vi "Initialize.vi"(8 "error in (no error)":errorcluster, 11 "Coins in":refnum<class "Coins.lvclass">) -> (0 "error out":errorcluster, 3 "Coins out":refnum<class "Coins.lvclass">)   [LabVIEW 2020, in "Coins.lvlib" / "Coins.lvclass"]
uses:
  Coins.lvclass
  Coins.lvclass/Coins.ctl
  Read Caller SubPanel.vi
  Read VI Refnum Actor Core.vi
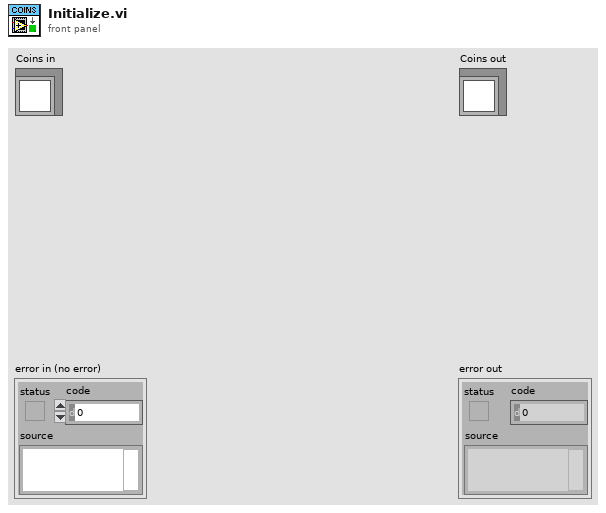
[diagram p1: front panel]
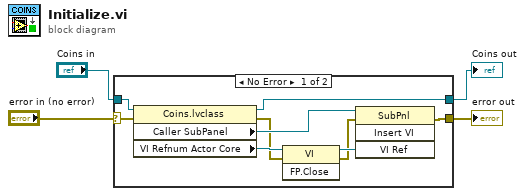
[diagram p0: block diagram]
diagram:
  n1 = case shown="No Error" "error in (no error)" {
    selector: "error in (no error)" -> [w11 w15]
    tunnel: [w9 w15] -> w3
    tunnel: [w12 w14] -> w1
    tunnel: "Coins in" -> [w13 w14]
    frame No Error {
      n2 = property class="Coins.lvclass"(reference=w13, error in=w11) -> (reference out=w12:refnum<class "Coins.lvclass">, error out=w6:errorcluster, "Caller SubPanel"=w10:refnum<vi>, "VI Refnum Actor Core"=w8:refnum<vi>)
      n3 = invoke class="VI" method="FP.Close"(reference=w8, error in=w6) -> (reference out=w7:refnum<vi>, error out=w5:errorcluster)  [unwired: 1 in, 1 out]
      n4 = invoke class="SubPnl" method="Insert VI"(reference=w10, error in=w5, "VI Ref"=w7) -> (error out=w9:errorcluster)  [unwired: 1 in, 3 out]
    }
    frame Error {
    }
  }
  "error out" <- w3
  "Coins out" <- w1
